vi "Close Visualizer.vi"(8 "error in (no error)":errorcluster, 11 "Visualizer ID":T1) -> (0 "error out":errorcluster)   [LabVIEW 2010, in "Visualizer.lvlib"]
doc: "Closes the visualizer window and disposes the visualizer ID. Any further VI calls using that ID will return an error."
uses:
  Visualizer.lvlib
  Visualizer Type ID.ctl
  Message.ctl
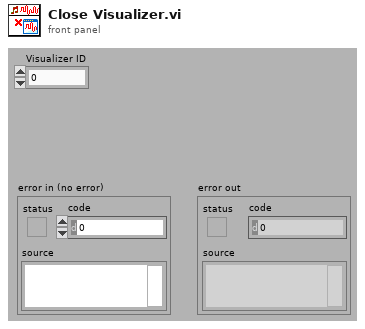
[diagram p1: front panel]
types:
  T1 = typedef "Visualizer.lvlib/Visualizer Type ID.ctl" = u32
  T2 = typedef "Visualizer.lvlib/Message.ctl" = cluster{"Command":string, "Data":variant}
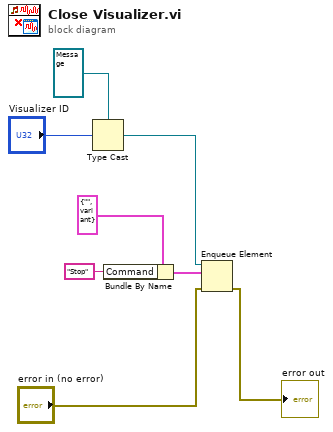
[diagram p0: block diagram]
diagram:
  n1 = Type Cast(type=refnum<queue> refnum ("queue out"), x="Visualizer ID") -> (*(type *) &x=w6:refnum<queue>)
  n2 = Bundle By Name(cluster=T2 {"Command"="", "Data"=variant} ("Message"), "Command"="Stop") -> (w1:T2)
  n3 = Enqueue Element(queue=w6, element=w1, error in (no error)="error in (no error)") -> (error out=→"error out":errorcluster)  [unwired: 1 in, 2 out]
